vi "Write DB Connection String.vi"(8 "error in (no error)":errorcluster, 10 "DB Connection String":string, 11 "CS++Factory in":refnum<class "CS++Factory.lvclass">) -> (0 "error out":errorcluster, 3 "CS++Factory out":refnum<class "CS++Factory.lvclass">)   [LabVIEW 2013, in "CS++BaseClasses.lvlib" / "CS++Factory.lvclass"]
doc: "Write DB connection String.\n\nCS++Factory uses a path to an ini-file. Derived factories may use the connection string for other stoarage media."
uses:
  CS++Factory.lvclass
  CS++Factory.lvclass/CS++Factory.ctl
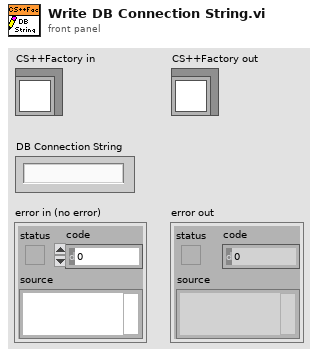
[diagram p1: front panel]
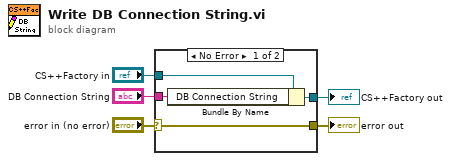
[diagram p0: block diagram]
diagram:
  n1 = case shown="No Error" "error in (no error)" {
    selector: "error in (no error)" -> [w9 w10]
    tunnel: [w9 w10] -> w4
    tunnel: [w7 w11] -> w2
    tunnel: "CS++Factory in" -> [w8 w11]
    tunnel: "DB Connection String" -> [w6 _]
    frame No Error {
      n2 = Bundle By Name(cluster=w8, "DB Connection String"=w6) -> (w7:refnum<class "CS++Factory.lvclass">)
    }
    frame Error {
    }
  }
  "error out" <- w4
  "CS++Factory out" <- w2
